vi "Dumb Dashboard Load.vi"(5 "section":string, 7 "refnum":T1, 9 "Name":string, 11 "Named Controls":T2) -> (2 "Found":bool)   [LabVIEW 2013]
uses:
  Named Control.ctl
  <vilib>/Utility/config.llb/Config Data RefNum.ctl
  <vilib>/Utility/config.llb/Read Key (Double).vi
  <vilib>/Utility/config.llb/Read Key (Boolean).vi
  <vilib>/Utility/config.llb/NI_LVConfig.lvlib
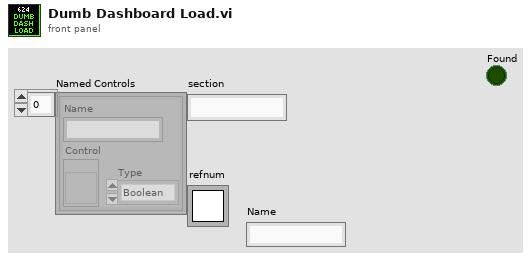
[diagram p1: front panel]
types:
  T1 = typedef "NI_LVConfig.lvlib/Config Data RefNum.ctl" = refnum<k1>
  T2 = typedef "Named Control.ctl" = cluster{"Name":string, "Control":refnum<vi>, "Type":enum16{"Boolean", "Double"}}[]
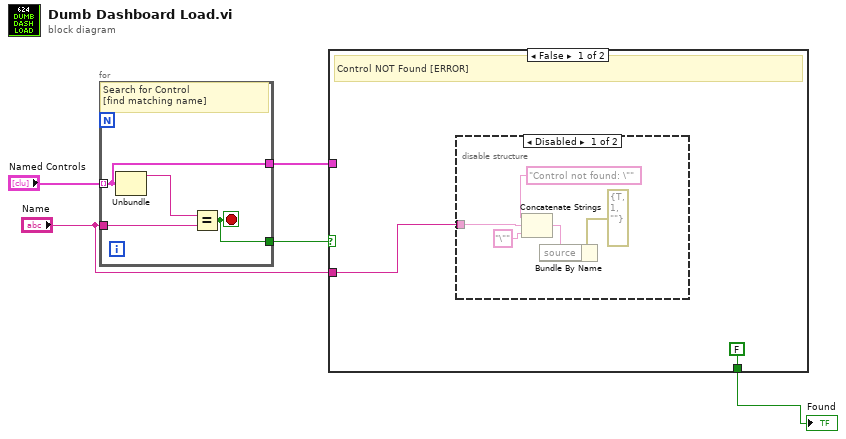
[diagram p0: block diagram]
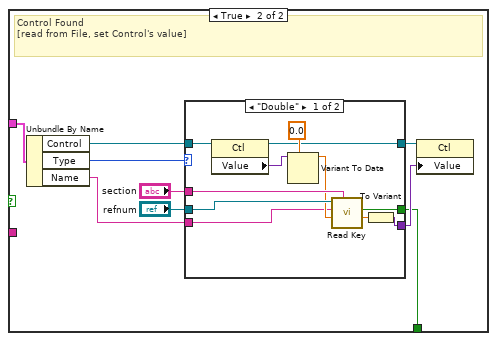
[diagram p3: hidden frame]
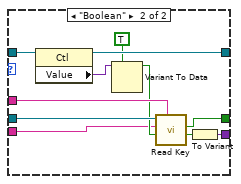
[diagram p4: hidden frame]
diagram:
  n1 = for {
    tunnel: "Named Controls" -> [w6] mode=indexing
    tunnel: [w9] -> w2
    tunnel: "Name" -> [w8]
    tunnel: [w6] -> w4
    stop <- w9 stop-if-true
    # "Search for Control\n[find matching name]"
    n2 = Unbundle(w6) -> ("Name"=w7:string)  [unwired: 2 out]
    n3 = Equal?(x=w7, y=w8) -> (x = y?=w9:bool)
  }
  n4 = case shown="False" w2 {
    tunnel: w4 -> [_ w21]
    tunnel: "Name" -> [w11 _]
    tunnel: [FALSE ("found?") w17] -> w1
    frame False {
      # "Control NOT Found [ERROR]"
      n5 = disable-structure shown="Disabled" {
        disable-tunnel: w11 -> [w12 _]
        frame Disabled {
          n6 = Concatenate Strings("Control not found: \"" ("string"), w12, "\"" ("string")) -> (w15:string)
          n7 = Bundle By Name(cluster=errorcluster {"status"=TRUE, "code"=1, "source"=""} ("error out"), "source"=w15) -> ()  [unwired: 1 out]
        }
        frame Enabled {
        }
      }
    }
    frame True {
      # "Control Found\n[read from File, set Control's value]"
      n8 = Unbundle By Name(w21) -> ("Control"=w20:refnum<vi>, "Type"=w19:enum16{"Boolean", "Double"}, "Name"=w18:string)
      n9 = case shown="\"Double\"" w19 {
        tunnel: "section" -> [w36 w47]
        tunnel: "refnum" -> [w35 w46]
        tunnel: [w30 w42] -> w23
        tunnel: w20 -> [w29 w41]
        tunnel: [w28 w40] -> w22
        tunnel: w18 -> [w27 w38]
        tunnel: [w26 w37] -> w17
        frame "Double" {
          n10 = property class="Ctl"(reference=w29) -> (reference out=w28:refnum<vi>, "Value"=w33:variant)  [unwired: 1 in, 1 out]
          n11 = Variant To Data(type=0.0, Variant=w33) -> (data=w32:dbl)  [unwired: 1 in, 1 out]
          n12 = call-poly <vilib>:"Read Key.vi"("section"=w36, "default value"=w32, "key"=w27, "refnum"=w35) -> ("value"=w31:dbl, "found?"=w26:bool)  [unwired: 4 in, 2 out]
          n13 = To Variant(anything=w31) -> (Variant=w30:variant)
        }
        frame "Boolean" {
          n14 = property class="Ctl"(reference=w41) -> (reference out=w40:refnum<vi>, "Value"=w45:variant)  [unwired: 1 in, 1 out]
          n15 = Variant To Data(type=TRUE, Variant=w45) -> (data=w44:bool)  [unwired: 1 in, 1 out]
          n16 = call-poly <vilib>:"Read Key.vi"("section"=w47, "default value"=w44, "key"=w38, "refnum"=w46) -> ("value"=w43:bool, "found?"=w37:bool)  [unwired: 4 in, 2 out]
          n17 = To Variant(anything=w43) -> (Variant=w42:variant)
        }
      }
      n18 = property class="Ctl"(reference=w22, "Value"=w23) -> ()  [unwired: 1 in, 2 out]
    }
  }
  "Found" <- w1
